vi "Compute Backplane Oversample Rate.vi"(3 "dt":sgl format="%.8e") -> (0 "start":dbl format="%.2f", 1 "Oversampling Rate (Hz)":sgl format="%.2f")   [LabVIEW 2017]
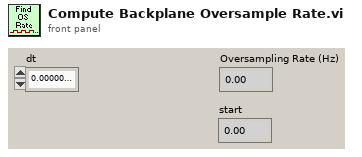
[diagram p1: front panel]
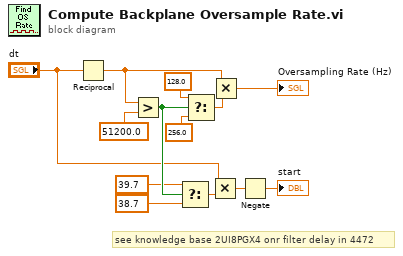
[diagram p0: block diagram]
diagram:
  # "see knowledge base 2UI8PGX4 onr filter delay in 4472"
  n1 = Reciprocal(x="dt") -> (1/x=w8:sgl)
  n2 = Greater?(x=w8, y=sgl 51200.0) -> (0:w7:bool)
  n3 = Select(t=39.7, s=w7, f=38.7) -> (s? t:f=w4:dbl)
  n4 = Select(t=sgl 128.0, s=w7, f=sgl 256.0) -> (s? t:f=w12:sgl)
  n5 = Multiply(x="dt", y=w4) -> (x*y=w2:dbl)
  n6 = Multiply(x=w8, y=w12) -> (x*y=→"Oversampling Rate (Hz)":sgl)
  n7 = Negate(x=w2) -> (-x=→"start":dbl)
